vi "acquisition_config.vi"(3 "error in":errorcluster, 4 "Timeserie config.":T1={"maximum value"=5.0, "minimum value"=-5.0, "Triggering level"=0.0, "Channel Trigger"=0, "Use Trigger?"=FALSE, "slope"=10280, "AVRG. TIMESERIE"=FALSE, "Fh(Hz)"=2.0, "N per cycle"=1024.0, "M cycles"=1.0} {"slope" items=["Rising"=10280, "Falling"=10171]; "Channel Trigger" items=["ai0", "ai1", "ai2", "ai3", "ai4", "ai5", "ai6", "ai7"]; "Triggering level" format="%0.5f"}, 5 "Analog In Channels":T2={"0"=TRUE, "1"=TRUE, "2"=TRUE, "3"=FALSE, "4"=FALSE, "5"=FALSE, "6"=FALSE, "7"=FALSE}) -> (0 "error out":errorcluster, 1 "Number of Samples indicator":i32=-1, 2 "task out":refnum<k21>)   [LabVIEW 2017]
uses:
  <vilib>/DAQmx/create/channels.llb/DAQmx Create Channel (AI-Voltage-Basic).vi
  <vilib>/DAQmx/configure/timing.llb/DAQmx Timing (Use Waveform).vi
  <vilib>/DAQmx/configure/trigger.llb/DAQmx Start Trigger (Analog Edge).vi
  <instrlib>/NI USB-6356/NI USB-6356.lvlib
panel:
  out "Sampling Frecuency indicator (Hz)":dbl
  # "Field monitor signal"
  # "Sensor signal AC"
  # "Sensor signal DC"
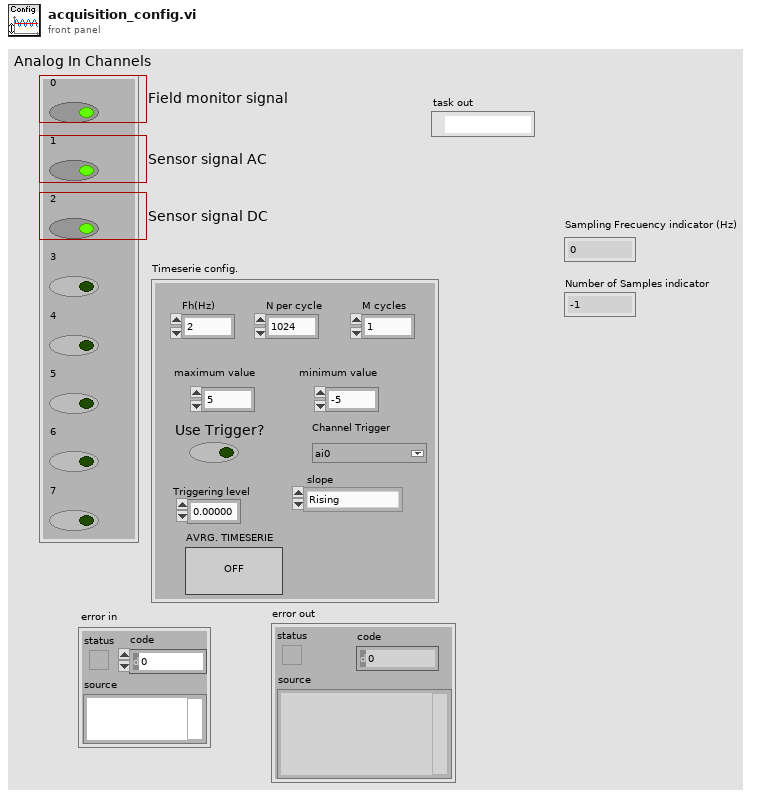
[diagram p1: front panel]
types:
  T1 = cluster{"maximum value":dbl, "minimum value":dbl, "Triggering level":dbl, "Channel Trigger":u16, "Use Trigger?":bool, "slope":i32, "AVRG. TIMESERIE":bool, "Fh(Hz)":dbl, "N per cycle":dbl, "M cycles":dbl}
  T2 = cluster{"0":bool, "1":bool, "2":bool, "3":bool, "4":bool, "5":bool, "6":bool, "7":bool}
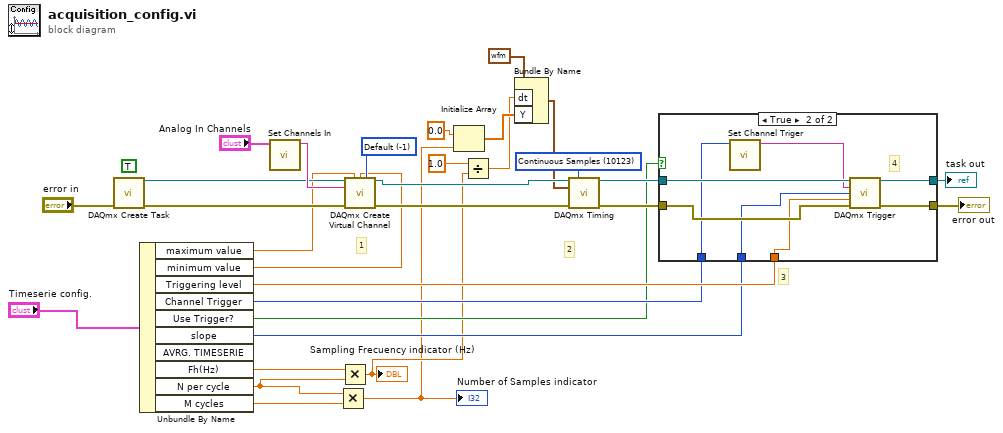
[diagram p0: block diagram]
diagram:
  (unwired) TRUE ("auto cleanup")
  w30 = 10123 items=["Finite Samples"=10178, "Continuous Samples"=10123, "Hardware Timed Single Point"=12522] ("sample mode")
  w31 = -1 items=["Default"=-1, "RSE"=10083, "Differential"=10106, "Pseudodifferential"=12529] ("output terminal configuration")
  # "3"
  # "2"
  # "1"
  n1 = call <vilib>:"DAQmx Create Task.vi"("error in"="error in") -> ("task out"=w16:refnum<k21>, "error out"=w15:errorcluster)  [unwired: 13 in]
  n2 = Unbundle By Name("Timeserie config.") -> ("maximum value"=w13:dbl, "minimum value"=w12:dbl, "Triggering level"=w11:dbl, "Channel Trigger"=w10:u16, "Use Trigger?"=w8:bool, "slope"=w9:i32, "Fh(Hz)"=w5:dbl, "N per cycle"=w4:dbl, "M cycles"=w3:dbl)  [unwired: 1 out]
  n3 = call <instrlib>:"Set Channels In.vi"("Analog In Channels"="Analog In Channels") -> ("String"=w18:string)  [unwired: 10 in]
  n4 = Multiply(x=w4, y=w3) -> (x*y=w1:dbl)
  "Number of Samples indicator" <- w1
  n5 = Multiply(x=w5, y=w4) -> (x*y=w2:dbl)
  "Sampling Frecuency indicator (Hz)" <- w2
  n6 = call-poly <vilib>:"DAQmx Create Virtual Channel.vi"("task in"=w16, "maximum value"=w13, "minimum value"=w12, "input terminal configuration"=w31, "physical channels"=w18, "error in"=w15) -> ("task out"=w29:refnum<k21>, "error out"=w25:errorcluster)  [unwired: 8 in]
  n7 = Initialize Array(0.0 ("element"), w1) -> (w26:dbl[])
  n8 = Divide(x=1.0, y=w2) -> (x/y=w23:dbl)
  n9 = Bundle By Name(cluster=waveform(dbl) {"t0"=timestamp(0 s since 1904-01-01), "dt"=0.001, "Y"=array[1000 elements]} ("signal out"), "dt"=w23, "Y"=w26) -> (w22:waveform(dbl))
  n10 = call-poly <vilib>:"DAQmx Timing.vi"("task/channels in"=w29, "sample mode"=w30, "waveform"=w22, "error in"=w25) -> ("task out"=w21:refnum<k21>, "error out"=w20:errorcluster)  [unwired: 10 in]
  n11 = case shown="True" w8 {
    tunnel: w21 -> [w33 w41]
    tunnel: w20 -> [w32 w38]
    tunnel: [w33 w40] -> w7
    tunnel: [w32 w39] -> w6
    tunnel: w11 -> [_ w36]
    tunnel: w10 -> [_ w35]
    tunnel: w9 -> [_ w34]
    frame False {
    }
    frame True {
      # "4"
      n12 = call <instrlib>:"Set Channel Triger.vi"("Channel Trigger"=w35) -> ("String Channel"=w37:string)  [unwired: 10 in]
      n13 = call-poly <vilib>:"DAQmx Trigger.vi"("task/channels in"=w41, "source"=w37, "slope"=w34, "level"=w36, "error in"=w38) -> ("task out"=w40:refnum<k21>, "error out"=w39:errorcluster)  [unwired: 9 in]
    }
  }
  "error out" <- w6
  "task out" <- w7
